vi "超标留样全局.vi"() -> ()   [LabVIEW 2016, in "德润超标留样.lvlib"]
panel:
  out "仪器状态":T1 {"仪器时间" format="%<%Y/%m/%d %H:%M:%S>T"; "门状态" items=["关闭", "打开"]; "采样模式" items=["定时留样"=1, "时间等比"=2, "同步留样"=3, "外控留样"=4, "超标留样"=5]; "工作进程" items=["停止中"=0, "启动延时"=1, "外置泵延时"=2, "管路润洗"=3, "管存"=4, "留样"=5, "出水管路排空"=6, "采水管路排空"=7, "待机"=13]; "工作状态" items=["停止", "运行", "系统初始化"]}
  in  "VISA resource name":refnum<visa-resource-name>="COM2" caption="VISA资源名称"
  in  "外控留样读取更新":bool
  out "外控留样":T2
  in  "读取更新":bool
  out "超标留样":T3={"当前瓶号："=0.0, "平行样："=0.0, "留样瓶数："=0.0, "每瓶次数："=0.0, "每次留样："=0.0, "时间间隔："=0.0, "COD联机："=2, "氨氮联机："=2, "4mA浓度："=0.0, "20mA浓度："=0.0, "超标浓度："=0.0, "4mA浓度："=0.0, "20mA浓度:"=0.0, "超标浓度："=0.0} {"COD联机：" items=["继电器"=1, "模拟输入"=2, "串口连接"=3]; "氨氮联机：" items=["继电器"=1, "模拟输入"=2, "串口连接"=3]}
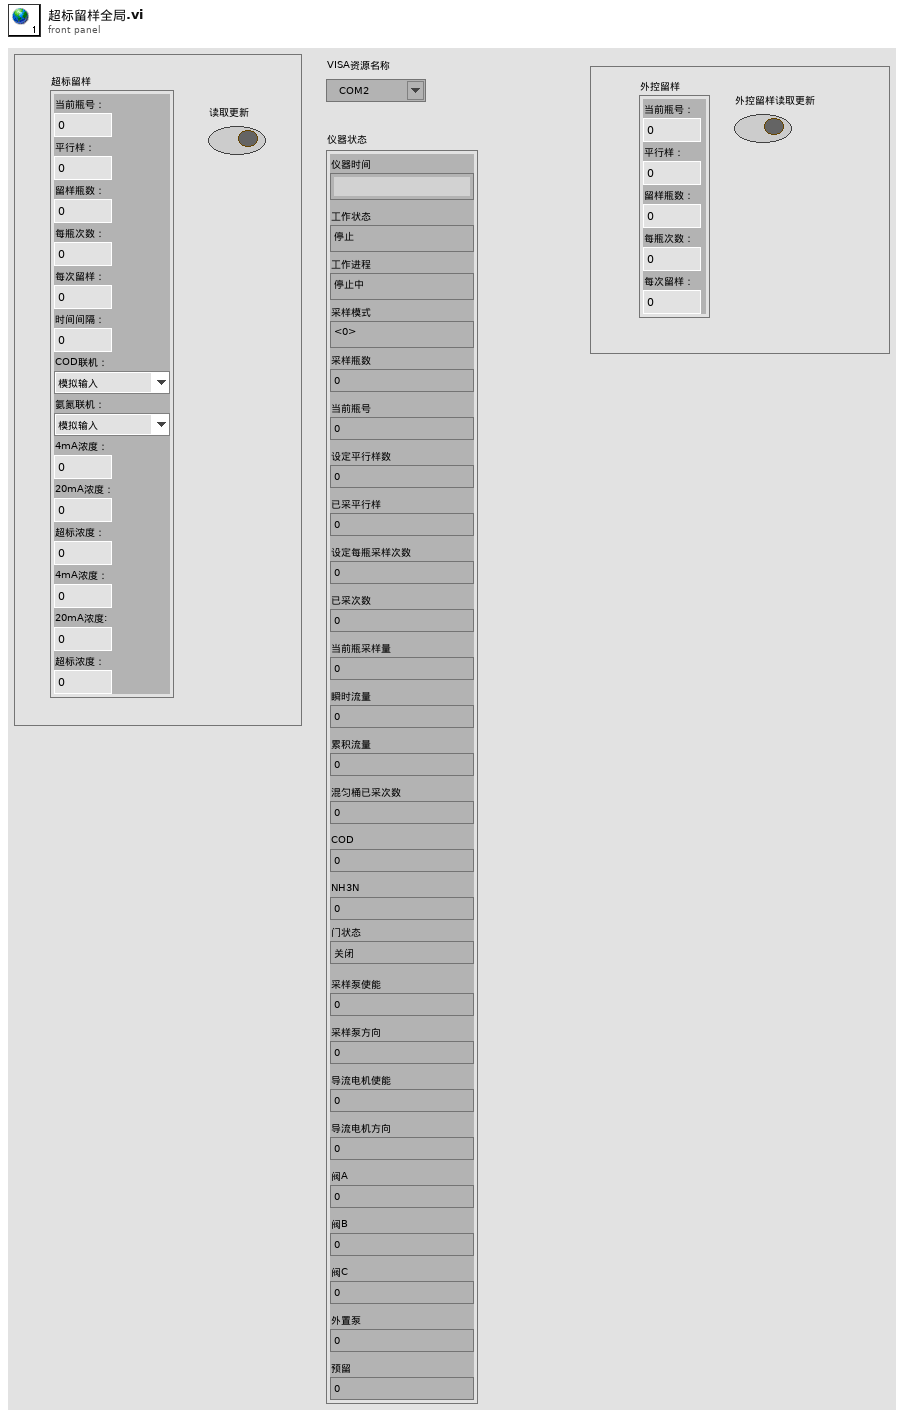
[diagram p1: front panel]
types:
  T1 = cluster{"仪器时间":timestamp, "工作状态":u16, "工作进程":u16, "采样模式":u16, "采样瓶数":dbl, "当前瓶号":dbl, "设定平行样数":dbl, "已采平行样":dbl, "设定每瓶采样次数":dbl, "已采次数":dbl, "当前瓶采样量":dbl, "瞬时流量":dbl, "累积流量":dbl, "混匀桶已采次数":dbl, "COD":dbl, "NH3N":dbl, "门状态":u16, "采样泵使能":dbl, "采样泵方向":dbl, "导流电机使能":dbl, "导流电机方向":dbl, "阀A":dbl, "阀B":dbl, "阀C":dbl, "外置泵":dbl, "预留":dbl}
  T2 = cluster{"当前瓶号：":dbl, "平行样：":dbl, "留样瓶数：":dbl, "每瓶次数：":dbl, "每次留样：":dbl}
  T3 = cluster{"当前瓶号：":dbl, "平行样：":dbl, "留样瓶数：":dbl, "每瓶次数：":dbl, "每次留样：":dbl, "时间间隔：":dbl, "COD联机：":u16, "氨氮联机：":u16, "4mA浓度：":dbl, "20mA浓度：":dbl, "超标浓度：":dbl, "4mA浓度：":dbl, "20mA浓度:":dbl, "超标浓度：":dbl}
diagram:
